vi "ClientSrv Server File Manipulation_srv.vi"(0 "method":T1=enum."list", 1 "new name":string, 5 "path":path, 7 "certificate":string, 9 "refnum in":refnum<file>, 11 "read amount":i32, 12 "data in":string, 13 "overwrite (F)":bool) -> (2 "directory":bool, 3 "last mod":timestamp, 4 "file names":string[](array[string]), 6 "directory names":string[](array[string]), 8 "length":i32, 10 "refnum out":refnum<file>, 14 "data out":string, 15 "error out":errorcluster)   [LabVIEW 2012]
doc: "Makes various file manipulations available remotely. When a relative path is specified, it is assumed to be relative to the resource base path. By doing all file manipulation through this one VI, the client-induced I/O load is pushed through this one bottleneck and thereby limited."
uses:
  typedefs/t_ClientSrv Server File Manipulation Methods.ctl
  typedefs/t_ClientSrv Access Levels.ctl
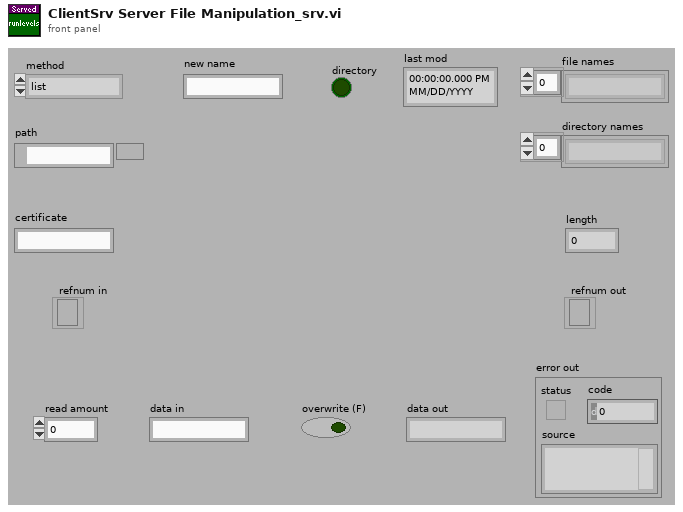
[diagram p1: front panel]
types:
  T1 = typedef "t_ClientSrv Server File Manipulation Methods.ctl" = enum16{"close", "list", "open", "new", "read", "write", "newdir", "info", "rename", "delete"}
  T2 = typedef "t_ClientSrv Access Levels.ctl" = enum16{"observer", "operator", "local"}
  T3 = enum16{"read/write", "read-only", "write-only", "write-only (truncate)"}
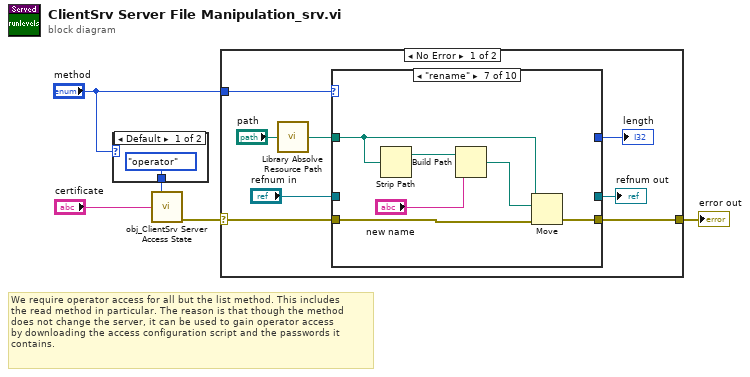
[diagram p0: block diagram]
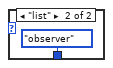
[diagram p2: hidden frame]
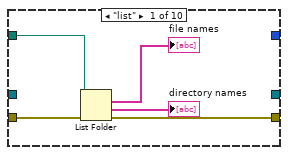
[diagram p3: hidden frame]
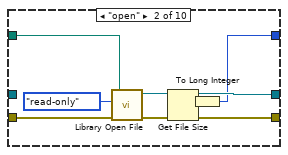
[diagram p4: hidden frame]
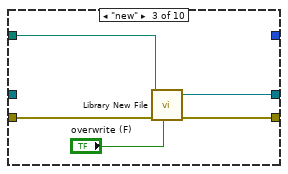
[diagram p5: hidden frame]
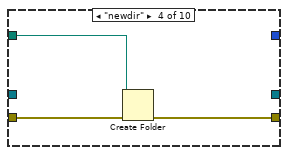
[diagram p6: hidden frame]
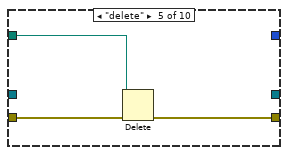
[diagram p7: hidden frame]
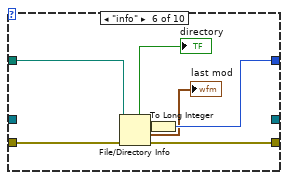
[diagram p8: hidden frame]
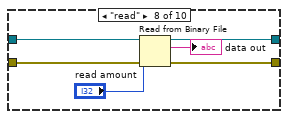
[diagram p9: hidden frame]
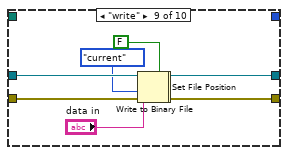
[diagram p10: hidden frame]
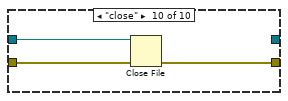
[diagram p11: hidden frame]
diagram:
  # "We require operator access for all but the list method. This includes\nthe read method in particular. The reason is that though the method\ndoes not change the server, it can be used to gain operator access\nby downloading the access configuration script and the passwords it\ncontains."
  n1 = case shown="Default" "method" {
    tunnel: [t_ClientSrv_Access_Levels."operator" ("access level") t_ClientSrv_Access_Levels."observer" ("access level")] -> w2
    frame Default {
    }
    frame "list" {
    }
  }
  n2 = call "obj_ClientSrv Server Access State.vi"("access level"=w2, "certificate in"="certificate") -> ("error out"=w3:errorcluster)  [unwired: 11 in, 2 out]
  n3 = case shown="No Error" w3 {
    selector: w3 -> [w12 w72]
    tunnel: [w14 w72] -> w4
    tunnel: "method" -> [w8 _]
    frame No Error {
      n4 = call "Library Absolve Resource Path.vi"("path in"="path") -> ("absolved path"=w13:path)  [unwired: 14 in]
      n5 = case shown="\"rename\"" w8 {
        tunnel: w12 -> [w20 w27 w34 w37 w40 w47 w53 w59 w68 w70]
        tunnel: [w19 w24 w33 w36 w39 w46 w52 w58 w67 w69] -> w14
        tunnel: w13 -> [w18 w29 w32 w35 w38 w45 w51 _ _ _]
        tunnel: [_ w23 w31 _ _ _ _ w56 w65 _] -> w11
        tunnel: "refnum in" -> [_ _ _ _ _ _ _ w57 w66 w71]
        tunnel: [_ w22 _ _ _ w44 _ _ _ _] -> w9
        frame "list" {
          n6 = List Folder(path=w18, error in=w20) -> (filenames=→"file names":string[], folder names=→"directory names":string[], error out=w19:errorcluster)  [unwired: 2 in, 1 out]
        }
        frame "open" {
          n7 = call "Library Open File.vi"("error in (no error)"=w27, "open mode (read/write)"=T3."read-only", "file path"=w29) -> ("error out"=w26:errorcluster, "refnum"=w25:refnum<file>)  [unwired: 3 in]
          n8 = Get File Size(file=w25, error in=w26) -> (refnum out=w23:refnum<file>, size (in bytes)=w21:i64, 0:w24:errorcluster)
          n9 = To Long Integer(number=w21) -> (32bit integer=w22:i32)
        }
        frame "new" {
          n10 = call "Library New File.vi"("overwrite (F)"="overwrite (F)", "error in (no error)"=w34, "file path"=w32) -> ("error out"=w33:errorcluster, "refnum"=w31:refnum<file>)  [unwired: 7 in]
        }
        frame "newdir" {
          n11 = Create Folder(path (use dialog)=w35, error in=w37) -> (error out=w36:errorcluster)  [unwired: 1 in, 2 out]
        }
        frame "delete" {
          n12 = Delete(path (use dialog)=w38, error in=w40) -> (error out=w39:errorcluster)  [unwired: 3 in, 2 out]
        }
        frame "info" {
          n13 = File/Directory Info(path=w45, error in=w47) -> (directory=→"directory":bool, size=w41:i64, last mod=→"last mod":timestamp, error out=w46:errorcluster)  [unwired: 3 out]
          n14 = To Long Integer(number=w41) -> (32bit integer=w44:i32)
        }
        frame "rename" {
          n15 = Strip Path(path=w51) -> (stripped path=w50:path)  [unwired: 1 out]
          n16 = Build Path(base path=w50, name or relative path="new name") -> (appended path=w48:path)
          n17 = Move(source path=w51, error in=w53, 10:w48) -> (error out=w52:errorcluster)  [unwired: 2 in, 2 out]
        }
        frame "read" {
          n18 = Read from Binary File(8:w59, 10:"read amount", 11:w57) -> (0:w58:errorcluster, 2:→"data out":string, 3:w56:refnum<file>)  [unwired: 3 in, 1 out]
        }
        frame "write" {
          n19 = Set File Position(refnum=w66, from (0:start)=enum16{"start", "end", "current"}."current" ("pos mode (0:2)"), error in=w68) -> (refnum out=w62:refnum<file>, error out=w61:errorcluster)  [unwired: 1 in]
          n20 = Write to Binary File(file (use dialog)=w62, data="data in", error in=w61, 5:FALSE ("prepend array or string size? (T)")) -> (refnum out=w65:refnum<file>, error out=w67:errorcluster)  [unwired: 2 in, 1 out]
        }
        frame "close" {
          n21 = Close File(refnum=w71, error in=w70) -> (error out=w69:errorcluster)  [unwired: 1 out]
        }
      }
      "length" <- w9
      "refnum out" <- w11
    }
    frame Error {
    }
  }
  "error out" <- w4
